vi "Day 6 - Tuning Trouble.vi"() -> ()   [LabVIEW 2020, in "AoC 2022.lvlib"]
uses:
  AoC 2022.lvlib
panel:
  out "Puzzle Part-2 Answer":string
  out "Puzzle Answer":string
  in  "Puzzle Input":string="mjqjpqmgbljsphdztnvjfqwrcgsmlb"
  # "Press Ctrl+M & Enter the Puzzle Input and run the VI"
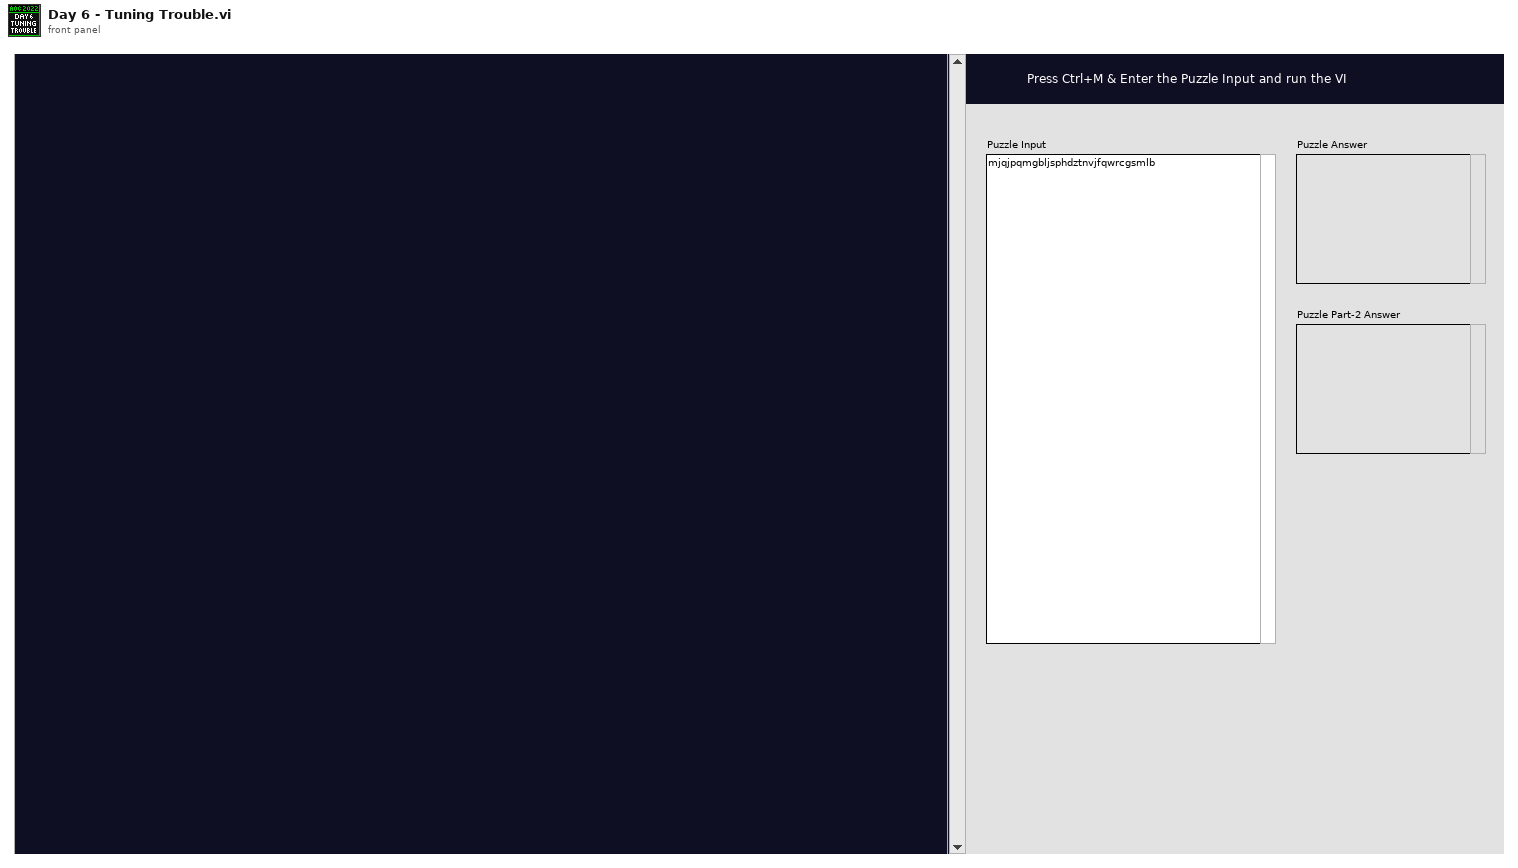
[diagram p1: front panel]
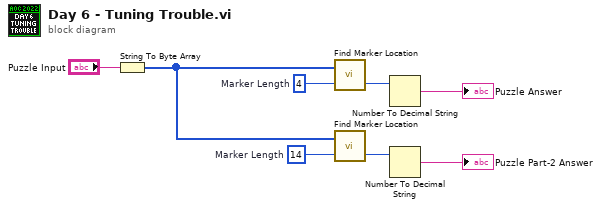
[diagram p0: block diagram]
diagram:
  w2 = 14  # Marker Length
  w7 = 4  # Marker Length
  n1 = String To Byte Array(string="Puzzle Input") -> (unsigned byte array=w3:u8[])
  n2 = call "Find Marker Location.vi"("Marker Length"=w7, "Datastream Buffer"=w3) -> ("Marker Appeared at"=w6:i32)  [unwired: 1 out]
  n3 = call "Find Marker Location.vi"("Marker Length"=w2, "Datastream Buffer"=w3) -> ("Marker Appeared at"=w1:i32)  [unwired: 1 out]
  n4 = Number To Decimal String(number=w6) -> (decimal integer string=→"Puzzle Answer":string)  [unwired: 1 in]
  n5 = Number To Decimal String(number=w1) -> (decimal integer string=→"Puzzle Part-2 Answer":string)  [unwired: 1 in]
